vi "SCMP - FPS reg.vi"(11 "FPS in":dbl) -> (3 "FPS out":dbl)   [LabVIEW 2014]
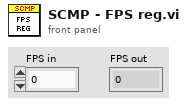
[diagram p1: front panel]
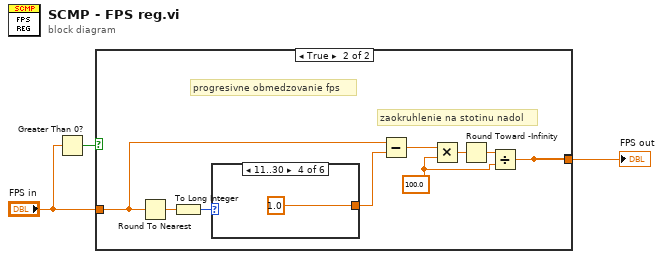
[diagram p0: block diagram]
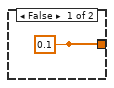
[diagram p2: hidden frame]
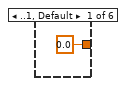
[diagram p3: hidden frame]
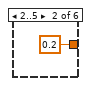
[diagram p4: hidden frame]
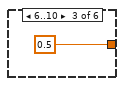
[diagram p5: hidden frame]
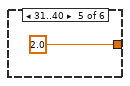
[diagram p6: hidden frame]
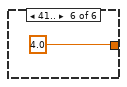
[diagram p7: hidden frame]
diagram:
  n1 = Greater Than 0?(x="FPS in") -> (x > 0?=w1:bool)
  n2 = case shown="True" w1 {
    tunnel: [w4 w7] -> _
    tunnel: "FPS in" -> [_ w5]
    tunnel: [w4 w7] -> w3
    frame False {
      w4 = 0.1
    }
    frame True {
      w9 = 100.0 ("y")
      # "zaokruhlenie na stotinu nadol"
      # "progresivne obmedzovanie fps"
      n3 = Round To Nearest(number=w5) -> (nearest integer value=w6:dbl)
      n4 = To Long Integer(number=w6) -> (32bit integer=w8:i32)
      n5 = case shown="11..30" w8 {
        tunnel: [0.0 0.2 0.5 1.0 2.0 4.0] -> w13
        frame ..1, Default {
        }
        frame 2..5 {
        }
        frame 6..10 {
        }
        frame 11..30 {
        }
        frame 31..40 {
        }
        frame 41.. {
        }
      }
      n6 = Subtract(x=w5, y=w13) -> (x-y=w12:dbl)
      n7 = Multiply(x=w12, y=w9) -> (x*y=w11:dbl)
      n8 = Round Toward -Infinity(1:w11) -> (0:w10:dbl)
      n9 = Divide(x=w10, y=w9) -> (x/y=w7:dbl)
    }
  }
  "FPS out" <- w3
